vi "ExManualCalibSave.vi"() -> ()   [LabVIEW 2010]
panel:
  in  "Full File Name to Write":path=path "C:/Program Files/SIToolKit/LabVIEW/Data Files/CalibHGArgon2.TIF"
  in  "stop":bool
  in  "Finished picking peaks":bool
  out "XY Graph":cluster{dbl[], "Array i32":i32[]}(graph)
  in  "Wavelength 3":dbl=576.96 format="%.2f"
  in  "Pixel 3":dbl=537.0 format="%.2f"
  in  "Wavelength 2":dbl=546.074 format="%.2f"
  in  "Pixel 2":dbl=485.0 format="%.2f"
  in  "Wavelength 1":dbl=435.833 format="%.2f"
  in  "Pixel 1":dbl=301.0 format="%.2f"
  out "error out":errorcluster
  in  "error in (no error)":errorcluster
  in  "FileType":u32=67174400
  in  "Full File Name to Read":path=path "C:/Program Files/SIToolKit/LabVIEW/Data Files/HG-ARGON.TIF"
  # "ExManualCalibSave.vi : this example shows how to do\na manual calibration. First select a file with data in\nit with know peaks (i.e. mercury lamp). then start VI.\nEnter pixel of peak with what wavelength peak should be.\nThis example does three peaks, but more can be used\nif available. Once all pixels and wavelengths have been\nentered then hit the finished button. The displahy will\nnow show a calibrated data with wavelength on the \nx axis. The cursor can be moved around to verify\nthe calibration. Hit stop button when done with calibration.\nUser may want to save calibration points in ascii file so that \nthese values can be used when collecting live data.\nThis example also saves the resulting calibrated data into a \nTIF file."
  # "File Types:\nSPE = 67371008\nTIF   = 67174400\nPMI  = 67436544"
  # "Note: currently only TIF files save the calibration too."
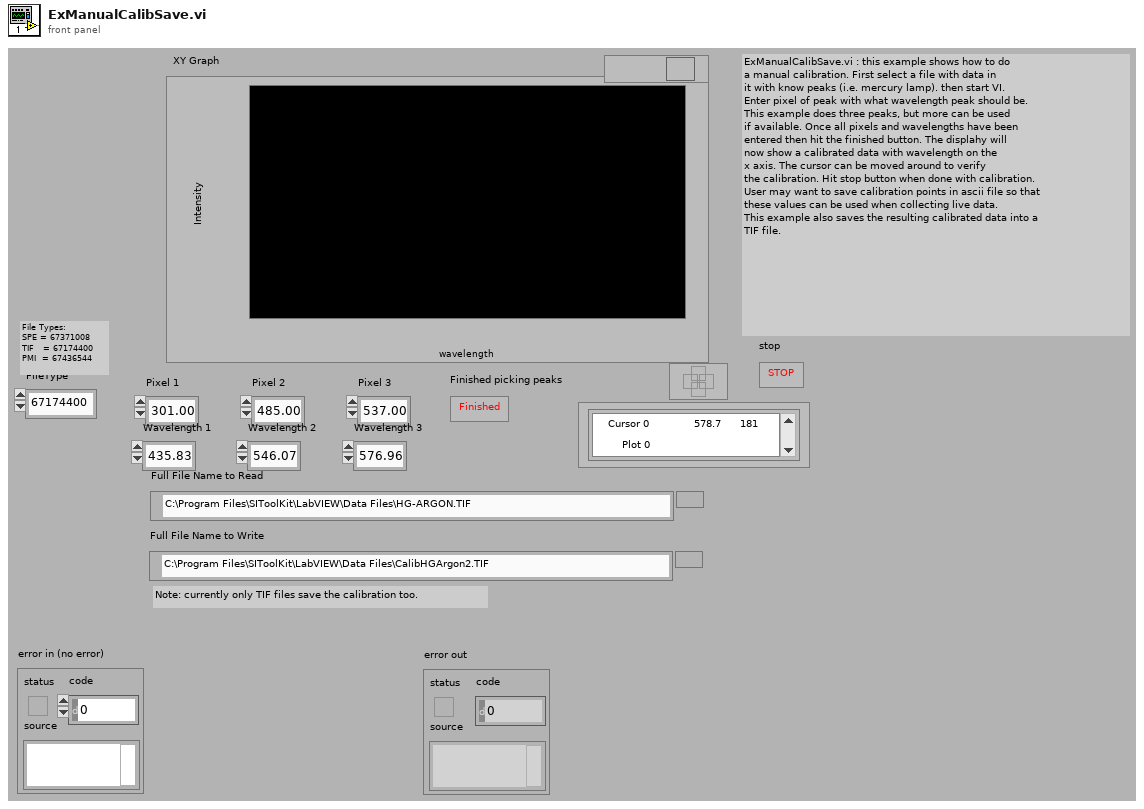
[diagram p1: front panel]
types:
  T1 = cluster{"total pairs":i32, "Order of\npolynominal":i32, "Units in\n4 is  wavelength in nm":i32, "Units out\n4 nm":i32, "Laser line wavelength in nm":dbl}
  T2 = cluster{"Calibrated Array":dbl[], "Array i32":i32[]}
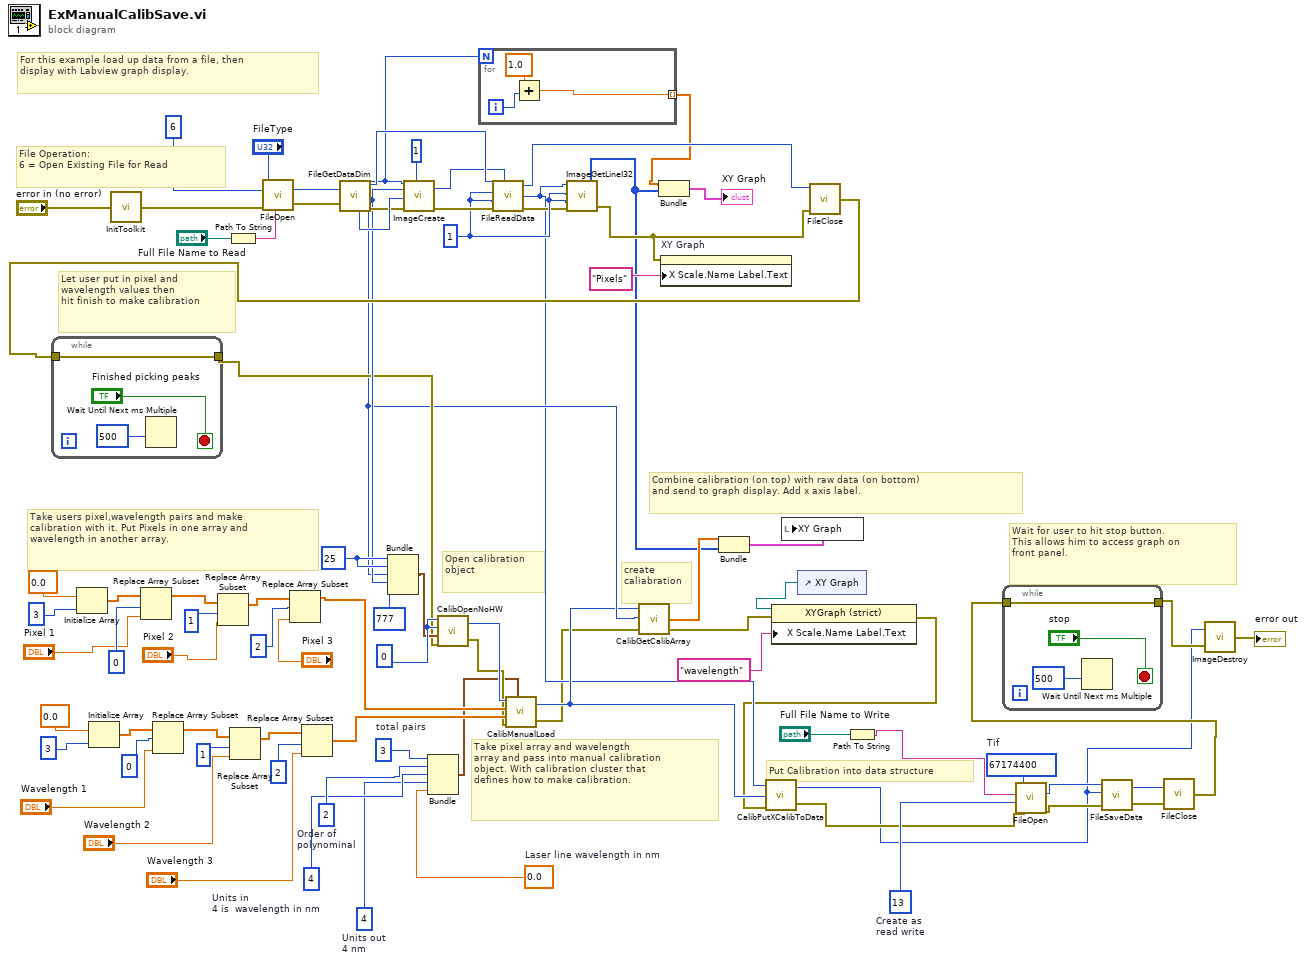
[diagram p0: block diagram]
diagram:
  w12 = 13  # Create as  read write
  w13 = 67174400  # Tif
  w35 = 0.0  # Laser line wavelength in nm
  w36 = 4  # Units out 4 nm
  w37 = 4  # Units in 4 is  wavelength in nm
  w38 = 2  # Order of polynominal
  w39 = 3  # total pairs
  w40 = 0
  w42 = 25
  w71 = 1
  # "Put Calibration into data structure"
  # "Wait for user to hit stop button.\nThis allows him to access graph on\nfront panel."
  # "Combine calibration (on top) with raw data (on bottom) \nand send to graph display. Add x axis label."
  # "create \ncaliabration"
  # "Take pixel array and wavelength \narray and pass into manual calibration \nobject. With calibration cluster that \ndefines how to make calibration."
  # "Open calibration\nobject"
  # "Take users pixel,wavelength pairs and make \ncalibration with it. Put Pixels in one array and\nwavelength in another array."
  # "Let user put in pixel and \nwavelength values then \nhit finish to make calibration"
  # "For this example load up data from a file, then\ndisplay with Labview graph display."
  # "File Operation:\n6 = Open Existing File for Read"
  n1 = Initialize Array(0.0, 3) -> (w59:dbl[])
  n2 = Initialize Array(0.0, 3) -> (w52:dbl[])
  n3 = call <userlib>:"InitToolkit.vi"("error in"="error in (no error)") -> ("error out"=w82:errorcluster)
  n4 = Replace Array Subset(array=w59, new element="Pixel 1", index=0) -> (w58:dbl[])
  n5 = Replace Array Subset(array=w52, new element="Wavelength 1", index=0) -> (w51:dbl[])
  n6 = Replace Array Subset(array=w58, new element="Pixel 2", index=1) -> (w57:dbl[])
  n7 = Path To String(path="Full File Name to Read") -> (string=w76:string)
  n8 = Replace Array Subset(array=w51, new element="Wavelength 2", index=1) -> (w50:dbl[])
  n9 = call <userlib>:"FileOpen.vi"("error in"=w82, "File Operations"=u32 6 ("File Operation"), "FileName"=w76, "File Type"="FileType") -> ("error out"=w80:errorcluster, "File Handle"=w79:u32)
  n10 = Replace Array Subset(array=w57, new element="Pixel 3", index=2) -> (w45:dbl[])
  n11 = Replace Array Subset(array=w50, new element="Wavelength 3", index=2) -> (w46:dbl[])
  n12 = call <userlib>:"FileGetDataDim.vi"("File Handle"=w79, "error in"=w80) -> ("Data Type"=w69:u32, "File Handle"=w74:u32, "X dim"=w24:u32, "Y dim"=w27:u32, "error out"=w68:errorcluster)  [unwired: 1 out]
  n13 = Bundle(w42, w42, "X dim"=w24, "Y dim"=w27, 777) -> (w26:cluster{i32, i32, "X dim":u32, "Y dim":u32, i32})  [unwired: 1 in]
  n14 = call <userlib>:"ImageCreate.vi"("X dimension"=w24, "Y dimension"=w27, "Data Type"=w69, "error in"=w68, "Number Of Frames"=1) -> ("Image Handle"=w73:u32, "error out"=w75:errorcluster)
  n15 = Bundle("total pairs"=w39, "Order of\npolynominal"=w38, "Units in\n4 is  wavelength in nm"=w37, "Units out\n4 nm"=w36, "Laser line wavelength in nm"=w35) -> (w34:T1)  [unwired: 1 in]
  n16 = for {
    N: w24 -> [_]
    tunnel: [w85] -> w67 mode=indexing
    i -> [w86]
    n17 = Add(x=1.0, y=w86) -> (x+y=w85:dbl)
  }
  n18 = call <userlib>:"FileReadData.vi"("File Handle"=w74, "Start Frame"=w71, "End Frame"=w71, "error in"=w75, "Image Handle"=w73) -> ("File Handle"=w72:u32, "Image Handle"=w15:u32, "error out"=w70:errorcluster)
  n19 = call <userlib>:"ImageGetLineI32.vi"("error in"=w70, "Z Position"=w71, "Y Position"=w71, "Data Handle"=w15) -> ("error out"=w64:errorcluster, "Array i32"=w18:i32[])  [unwired: 1 out]
  n20 = Bundle(w67, "Array i32"=w18) -> (→"XY Graph":cluster{dbl[], "Array i32":i32[]})  [unwired: 1 in]
  n21 = property on="XY Graph" class="XYGraph (strict)"(error in=w64, "X Scale.Name Label.Text"="Pixels") -> ()  [unwired: 1 in, 2 out]
  n22 = control-ref of="XY Graph"() -> (w21:refnum<vi>)
  n23 = call <userlib>:"FileClose.vi"("error in"=w64, "File Handle"=w72) -> ("error out"=w63:errorcluster)
  n24 = while {
    tunnel: w63 -> [w89]
    tunnel: [w89] -> w25
    stop <- "Finished picking peaks" stop-if-true
    n25 = Wait Until Next ms Multiple(millisecond multiple=500) -> ()  [unwired: 1 out]
  }
  n26 = call <userlib>:"CalibOpenNoHW.vi"("error in"=w25, "Data Info"=w26, "Calibration Type"=w40, "Calibration Device ID"=w40) -> ("error out"=w43:errorcluster, "Calibration Handle"=w44:u32)
  n27 = call <userlib>:"CalibManualLoad.vi"("Calibration Handle"=w44, "Pixel Array"=w45, "Wavelength Array"=w46, "error in (no error)"=w43, "Calibration Values"=w34) -> ("Calibration Handle"=w16:u32, "error out"=w5:errorcluster)
  n28 = call <userlib>:"CalibGetCalibArray.vi"("error in"=w5, "Array Size"=w24, "Calibration Handle"=w16) -> ("error out"=w22:errorcluster, "Calibrated Array"=w19:dbl[])  [unwired: 1 out]
  n29 = Bundle("Calibrated Array"=w19, "Array i32"=w18) -> (w23:T2)  [unwired: 1 in]
  n30 = property on="Property Node" class="XYGraph (strict)"(reference=w21, error in=w22, "X Scale.Name Label.Text"="wavelength") -> (error out=w6:errorcluster)  [unwired: 1 out]
  n31 = call <userlib>:"CalibPutXCalibToData.vi"("error in (no error)"=w6, "Calibration Handle"=w16, "Data Handle"=w15) -> ("error out"=w11:errorcluster, "Data Handle"=w2:u32)
  n32 = local write "XY Graph"(w23) -> ()
  n33 = Path To String(path="Full File Name to Write") -> (string=w14:string)
  n34 = call <userlib>:"FileOpen.vi"("error in"=w11, "File Operations"=w12, "FileName"=w14, "File Type"=w13) -> ("error out"=w10:errorcluster, "File Handle"=w9:u32)
  n35 = call <userlib>:"FileSaveData.vi"("error in"=w10, "Image Handle"=w2, "File Handle"=w9) -> ("error out"=w8:errorcluster, "File Handle"=w7:u32)
  n36 = call <userlib>:"FileClose.vi"("error in"=w8, "File Handle"=w7) -> ("error out"=w4:errorcluster)
  n37 = while {
    tunnel: w4 -> [w91]
    tunnel: [w91] -> w3
    stop <- "stop" stop-if-true
    n38 = Wait Until Next ms Multiple(millisecond multiple=500) -> ()  [unwired: 1 out]
  }
  n39 = call <userlib>:"ImageDestroy.vi"("error in"=w3, "Data handle"=w2) -> ("error out"=→"error out":errorcluster)
